vi "Main_SubVI_Sort Comment.vi"(8 "Error In":errorcluster, 9 "Data":i32, 10 "Register  Address":i32, 11 "Axis Number":T1 items=["X"=1, "Y"=2, "Z"=3, "Rotation"=4]) -> (0 "Error Out":errorcluster, 3 "Command":string)   [LabVIEW 2015]
uses:
  Control/Control_Axis Number.ctl
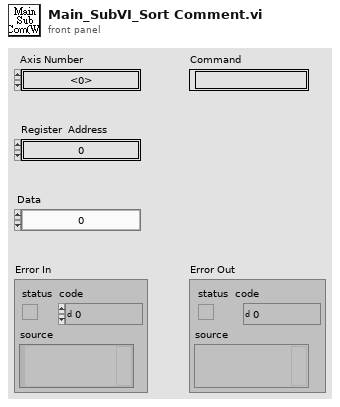
[diagram p1: front panel]
types:
  T1 = typedef "Control_Axis Number.ctl" = u16
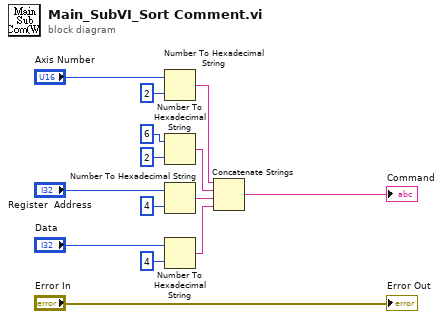
[diagram p0: block diagram]
diagram:
  n1 = Number To Hexadecimal String(1:i16 2 ("width (-)"), 2:"Axis Number") -> (0:w6:string)
  n2 = Number To Hexadecimal String(1:i16 2 ("width (-)"), 2:6 ("number")) -> (0:w5:string)
  n3 = Number To Hexadecimal String(1:i16 4 ("width (-)"), 2:"Register  Address") -> (0:w4:string)
  n4 = Number To Hexadecimal String(1:i16 4 ("width (-)"), 2:"Data") -> (0:w2:string)
  n5 = Concatenate Strings(w6, w5, w4, w2) -> (→"Command":string)
  "Error Out" <- "Error In"
